vi "SECoP-getStoredCommand.vi"(8 "error in (no error)":errorcluster, 11 "DLL path (in)":T3) -> (0 "error out":errorcluster, 1 "SECoP_data":T1 {"ptr64" format="%.0x"; "ptr32" format="%.0x"}, 2 "command/parameter path":string, 3 "DLL path (out)":T3, 4 "action":T2, 5 "command id":u64)   [LabVIEW 2023, in "SECoP.lvlib"]
doc: "Call <b>\"SECoP-getStoredCommand.vi\"</b> regulary to check, if there is something to do for any accessible. If yes, it will return successfully with an id, what to do, a parameter/command name and new set value or argument.\n\n<b>DLL path</b> input and output of cluster from \"SECoP-Initialize.vi\"\n<b>command id</b> on match: command id for \"SECoP-putCommandAnswer.vi\"\n<b>action id</b> on match: action id to handle\n<b>command/parameter path</b> on match: full name of accessible\n<b>SECoP_data</b> on match with change or do: input data from SECoP-client"
uses:
  SECoP.lvlib
  SECoP-libraries.ctl
  SECoP-action.ctl
  SECoP-data/SECoP-data.ctl
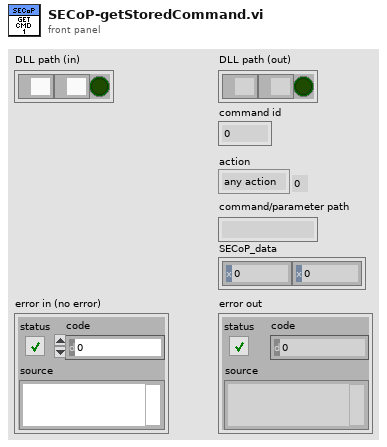
[diagram p1: front panel]
types:
  T1 = typedef "SECoP.lvlib/SECoP-data.ctl" = cluster{"ptr32":u32, "ptr64":u64}
  T2 = typedef "SECoP.lvlib/SECoP-action.ctl" = enum32{"any action", "read", "change", "do cmd"}
  T3 = typedef "SECoP.lvlib/SECoP-libraries.ctl" = cluster{"serverDLL":path, "variantDLL":path, "cleanup_mode":bool}
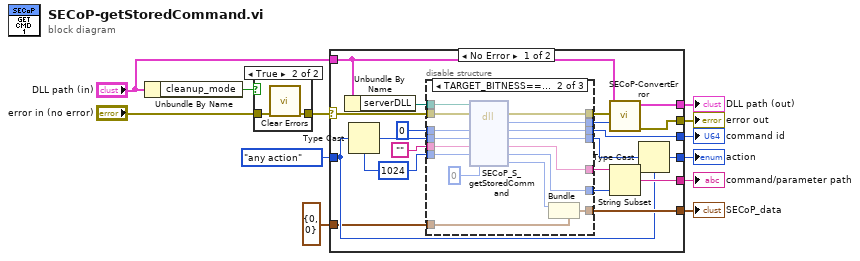
[diagram p0: block diagram]
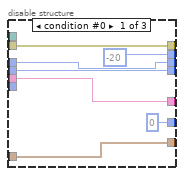
[diagram p3: hidden frame]
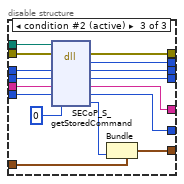
[diagram p4: hidden frame]
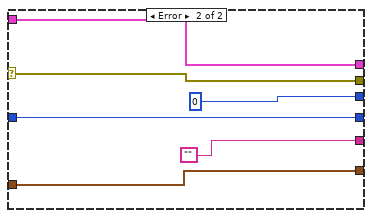
[diagram p5: hidden frame]
diagram:
  n1 = Unbundle By Name("DLL path (in)") -> ("cleanup_mode"=w8:bool)
  n2 = case shown="True" w8 {
    tunnel: "error in (no error)" -> [w13 w15]
    tunnel: [w13 w14] -> w6
    frame False {
    }
    frame True {
      n3 = call <vilib>:"Clear Errors.vi"("error in (no error)"=w15) -> ("error out"=w14:errorcluster)  [unwired: 5 in, 1 out]
    }
  }
  n4 = case shown="No Error" w6 {
    selector: w6 -> [w33 w79]
    tunnel: "DLL path (in)" -> [w17 w80]
    tunnel: [w34 w80] -> w12
    tunnel: [w35 w79] -> w11
    tunnel: [w26 i64 0 ("id")] -> w10
    tunnel: [w23 w77] -> w4
    tunnel: [w24 ""] -> w9
    tunnel: SECoP-action."any action" ("SECoP_action") -> [w21 w77]
    tunnel: [w22 w75] -> w2
    tunnel: T1 {"ptr32"=0, "ptr64"=0} ("SECoP_data") -> [w18 w75]
    frame No Error {
      w19 = 1024 ("parameter size")
      n5 = Unbundle By Name(w17) -> ("serverDLL"=w16:path)
      n6 = Type Cast(type=w19, x=w21) -> (*(type *) &x=w20:i32)
      n7 = disable-structure shown="TARGET_BITNESS==32" {
        disable-tunnel: w33 -> [w42 w58 w69]
        disable-tunnel: w16 -> [_ w57 w74]
        disable-tunnel: [w42 w56 w68] -> w32
        disable-tunnel: [-20 ("return type") w55 w67] -> w31
        disable-tunnel: u64 0 ("id") -> [w39 w54 w70]
        disable-tunnel: "" -> [w37 w53 w72]
        disable-tunnel: w19 -> [_ w52 w73]
        disable-tunnel: [0 ("parameter size") w51 w63] -> w28
        disable-tunnel: [w37 w50 w64] -> w27
        disable-tunnel: [w39 w49 w66] -> w26
        disable-tunnel: [w38 w48 w65] -> w25
        disable-tunnel: w20 -> [w38 w47 w71]
        disable-tunnel: [w40 w46 w60] -> w22
        disable-tunnel: w18 -> [w40 w45 w62]
        frame condition #0 {
        }
        frame condition #1 {
          n8 = dll-call lib="Z:/Praktische Aufgaben/SECoP-LabVIEW2015/32bit/SECoP32.dll" fn="SECoP_S_getStoredCommand"(path in=w57, error in=w58, "id"=w54, "command"=w47, "parameter"=w53, "parameter size"=w52, "value"=u32 0) -> (error out=w56:errorcluster, "return type"=w55:i32, "id"=w49:u64, "command"=w48:i32, "parameter"=w50:string, "parameter size"=w51:i32, "value"=w44:u32)  [unwired: 1 in, 1 out]
          n9 = Bundle(cluster=w45, "ptr32"=w44) -> (w46:T1)  [unwired: 1 in]
        }
        frame condition #2 (active) {
          n10 = dll-call lib="Z:/Praktische Aufgaben/SECoP-LabVIEW2015/32bit/SECoP32.dll" fn="SECoP_S_getStoredCommand"(path in=w74, error in=w69, "id"=w70, "command"=w71, "parameter"=w72, "parameter size"=w73, "value"=u64 0) -> (error out=w68:errorcluster, "return type"=w67:i32, "id"=w66:u64, "command"=w65:i32, "parameter"=w64:string, "parameter size"=w63:i32, "value"=w61:u64)  [unwired: 1 in, 1 out]
          n11 = Bundle(cluster=w62, "ptr64"=w61) -> (w60:T1)  [unwired: 1 in]
        }
      }
      n12 = call "SECoP-ConvertError.vi"("return code"=w31, "error in (no error)"=w32, "DLL path (in)"=w17) -> ("error out"=w35:errorcluster, "DLL path (out)"=w34:T3)  [unwired: 7 in]
      n13 = String Subset(string=w27, length (rest)=w28) -> (substring=w24:string)  [unwired: 1 in]
      n14 = Type Cast(type=w21, x=w25) -> (*(type *) &x=w23:T2)
    }
    frame Error {
    }
  }
  "DLL path (out)" <- w12
  "error out" <- w11
  "command/parameter path" <- w9
  "command id" <- w10
  "action" <- w4
  "SECoP_data" <- w2
